vi "Voltage K24xx Coarse.vi"() -> ()   [LabVIEW 2020]
panel:
  out "Voltage K24xx Coarse":dbl
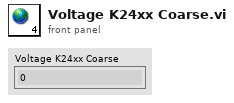
[diagram p1: front panel]
diagram:
